vi "Fit complex bg one.vi"(9 "Initial parameters":dbl[](array[numeric])=[188.484, 0.01, 0.00126452, 2.4, 1.1376494443646765, -0.8104040332703796], 10 "Z":cdb[](array[numeric]), 11 "X":dbl[](array[numeric])) -> ()   [LabVIEW 2016]
uses:
  <vilib>/gmath/NumericalOptimization/Nonlinear Curve Fit LM bound.vi
  <vilib>/gmath/NI_Gmath.lvlib
panel:
  out "residue":dbl
  in  "Bounds":T1={"parameter minimum"=[1.0, 1.0, 0.01, -0.1, -5.0, -5.0], "parameter maximum"=[20000000.0, 200.0, 100.0, 6.3, 5.0, 5.0]}
  out "Weight":dbl[](graph)
  out "best fit parameters":dbl[](array[numeric])
  out "number of function calls":i32
  in  "termination":cluster{"max iteration":i32, "tolerance":dbl}={"max iteration"=200, "tolerance"=1e-08}
  out "Fit":cluster{"X":dbl[], "best nonlinear fit":dbl[]}[](graph)
  # "F0\nG\nA\nP\nX\nY"
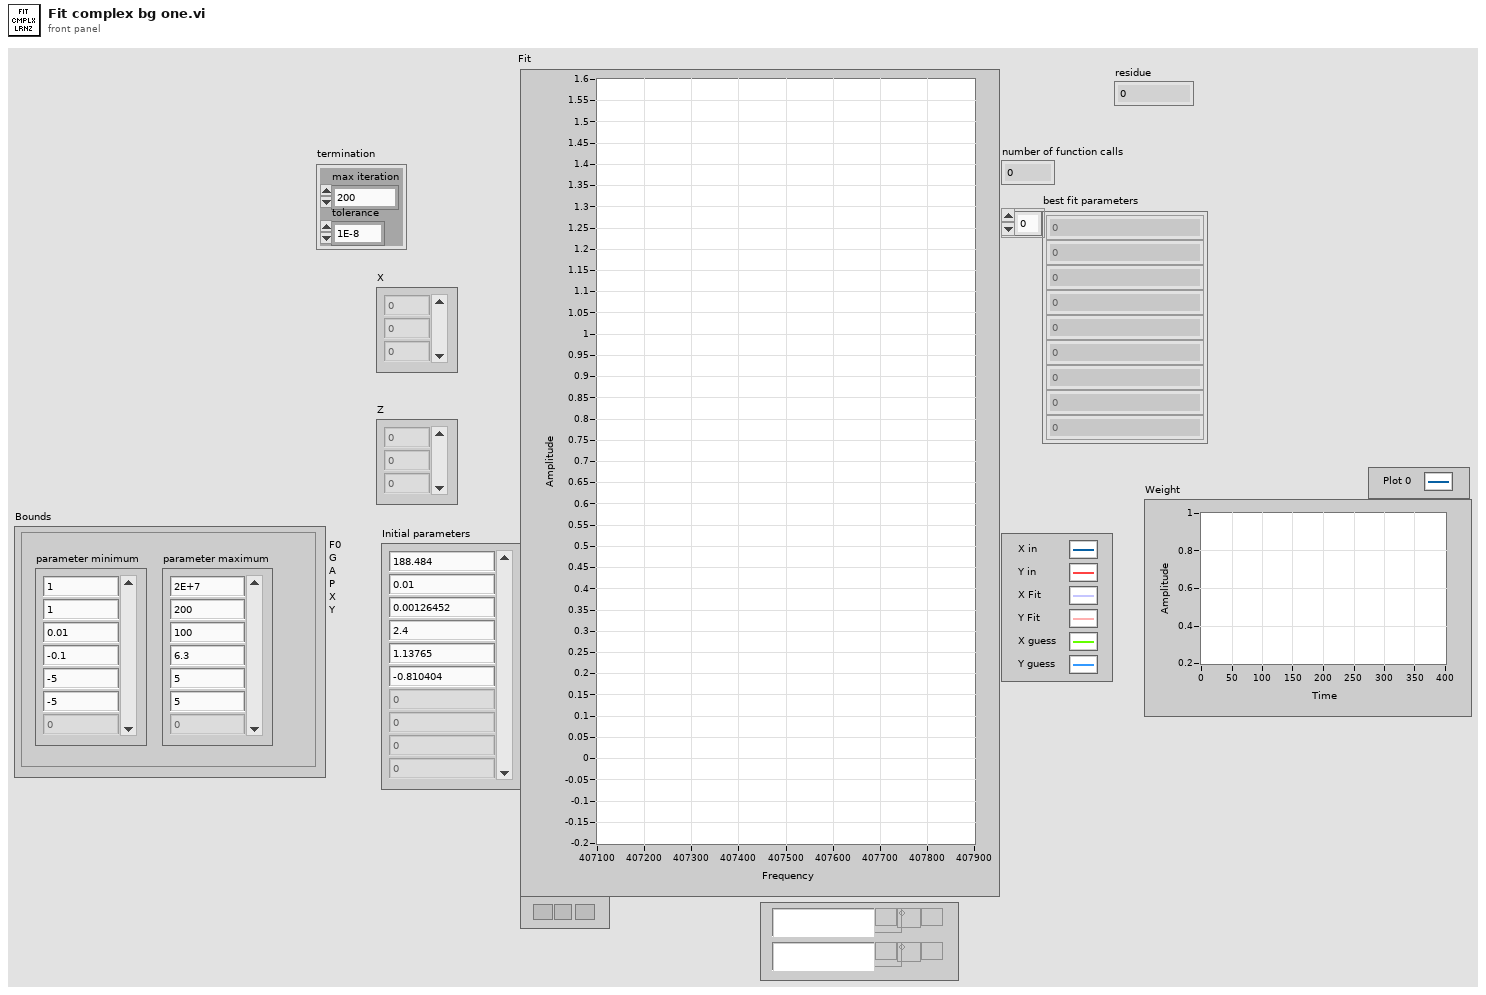
[diagram p1: front panel]
types:
  T1 = cluster{"parameter minimum":dbl[], "parameter maximum":dbl[]}
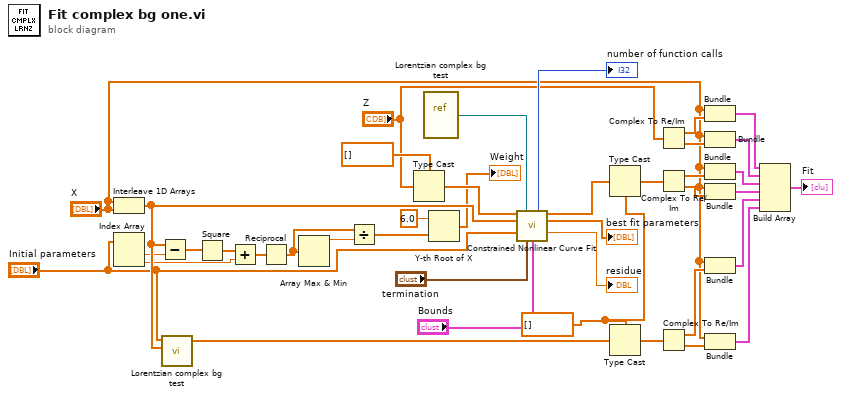
[diagram p0: block diagram]
diagram:
  w19 = cdb[] []
  n1 = Interleave 1D Arrays("X", "X") -> (w14:dbl[])
  n2 = Index Array(array="Initial parameters") -> (element #1=w12:dbl, element #2=w9:dbl)  [unwired: 2 in]
  n3 = Subtract(x=w14, y=w12) -> (x-y=w11:dbl[])
  n4 = call "Lorentzian complex bg test.vi"("X"=w14, "a"="Initial parameters") -> ("f(X,a)"=w21:dbl[])  [unwired: 2 in, 2 out]
  n5 = Square(x=w11) -> (x^2=w10:dbl[])
  n6 = Add(x=w10, y=w9) -> (x+y=w8:dbl[])
  n7 = Reciprocal(x=w8) -> (1/x=w7:dbl[])
  n8 = Array Max & Min(array=w7) -> (max value=w6:dbl)  [unwired: 3 out]
  n9 = Divide(x=w7, y=w6) -> (x/y=w3:dbl[])
  n10 = Type Cast(type=dbl[] [], x="Z") -> (*(type *) &x=w33:dbl[])
  n11 = vi-ref "Lorentzian complex bg test.vi"() -> (w40:refnum<vi>)
  n12 = Y-th Root of X(1:w3, 2:6.0) -> (0:→"Weight":dbl[])
  n13 = call-poly <vilib>:"Constrained Nonlinear Curve Fit.vi"("Y"=w33, "f(x,a)"=w40, "X"=w14, "initial parameters"="Initial parameters", "termination"="termination", "parameter bounds"="Bounds") -> ("number of function calls"=→"number of function calls":i32, "best nonlinear fit"=w31:dbl[], "best fit parameters"=→"best fit parameters":dbl[], "residue"=→"residue":dbl)  [unwired: 4 in, 2 out]
  n14 = Type Cast(type=w19, x=w31) -> (*(type *) &x=w25:cdb[])
  n15 = Type Cast(type=w19, x=w21) -> (*(type *) &x=w20:cdb[])
  n16 = Complex To Re/Im(x + iy="Z") -> (x=w29:dbl[], y=w28:dbl[])
  n17 = Complex To Re/Im(x + iy=w25) -> (x=w23:dbl[], y=w24:dbl[])
  n18 = Complex To Re/Im(x + iy=w20) -> (x=w18:dbl[], y=w16:dbl[])
  n19 = Bundle("X"="X", w29) -> (w27:cluster{"X":dbl[], dbl[]})  [unwired: 1 in]
  n20 = Bundle("X"="X", w28) -> (w26:cluster{"X":dbl[], dbl[]})  [unwired: 1 in]
  n21 = Bundle("X"="X", w23) -> (w22:cluster{"X":dbl[], dbl[]})  [unwired: 1 in]
  n22 = Bundle("X"="X", w24) -> (w39:cluster{"X":dbl[], dbl[]})  [unwired: 1 in]
  n23 = Bundle("X"="X", w18) -> (w34:cluster{"X":dbl[], dbl[]})  [unwired: 1 in]
  n24 = Bundle("X"="X", w16) -> (w15:cluster{"X":dbl[], dbl[]})  [unwired: 1 in]
  n25 = Build Array(w27, w26, w22, w39, w34, w15) -> (→"Fit":cluster{"X":dbl[], dbl[]}[])
